vi "OCR_Determine Line bit array.vi"(8 "Error":errorcluster, 9 "Body Rect Array":T2[](array[typedef]), 11 "Border Removed":T6) -> (0 "Error Out":errorcluster, 3 "Text Out":T1[](array[typedef]), 4 "Status Of Each Line Out":bool[](array[boolean]))   [LabVIEW 2009]
uses:
  Controls/Array/Color Box Array_2D Icon Viewer.ctl
  Controls/Cluster/Cluster_Text Rect.ctl
  Controls/Cluster/Cluster_Region info.ctl
  Controls/Cluster/Cluster_Top Left position.ctl
  Controls/Cluster/Cluster_Text Color Set.ctl
  Controls/String_Picture/STRING_Line Display.ctl
  Controls/Cluster/Cluster_Bit array and line status.ctl
  Controls/String_Picture/String Char Normal.ctl
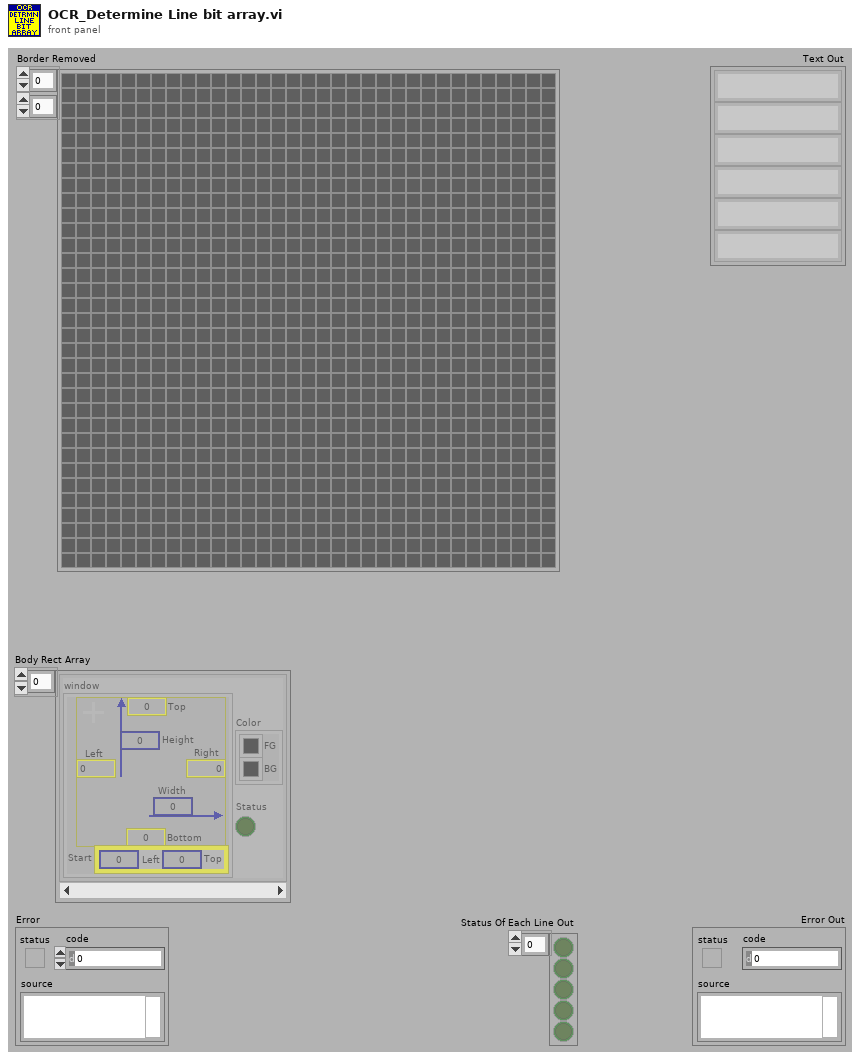
[diagram p1: front panel]
types:
  T1 = typedef "STRING_Line Display.ctl" = string
  T2 = typedef "Cluster_Text Rect.ctl" = cluster{"window":T3, "Color":T5, "Status":bool}
  T3 = typedef "Cluster_Region info.ctl" = cluster{"Left":i32, "Top":i32, "Right":i32, "Bottom":i32, "Width":u32, "Height":u32, "Start":T4}
  T4 = typedef "Cluster_Top Left position.ctl" = cluster{"Left":i32, "Top":i32}
  T5 = typedef "Cluster_Text Color Set.ctl" = cluster{"BG":u32, "FG":u32}
  T6 = typedef "Color Box Array_2D Icon Viewer.ctl" = u32[][]
  T7 = typedef "Cluster_Bit array and line status.ctl" = cluster{"Char Array":T8[], "Status":bool}
  T8 = typedef "String Char Normal.ctl" = string
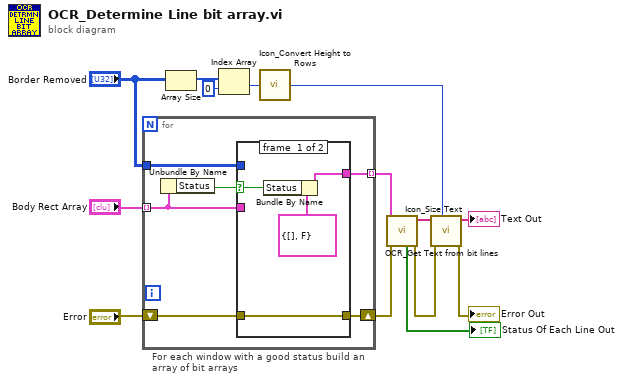
[diagram p0: block diagram]
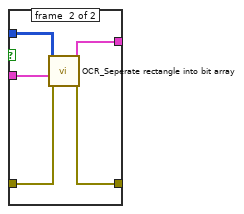
[diagram p2: hidden frame]
diagram:
  n1 = for "For each window with a good status build an array of bit arrays" {
    tunnel: [w17] -> w12 mode=indexing
    tunnel: "Body Rect Array" -> [w15] mode=indexing
    shift-right: [w19] -> w11
    shift-left: "Error" -> [w20]
    tunnel: "Border Removed" -> [w18]
    n2 = Unbundle By Name(w15) -> ("Status"=w16:bool)
    n3 = case shown="False" w16 {
      selector: w16 -> [w21 _]
      tunnel: w20 -> [w24 w29]
      tunnel: [w24 w28] -> w19
      tunnel: w18 -> [_ w27]
      tunnel: w15 -> [_ w26]
      tunnel: [w22 w25] -> w17
      frame #0 {
        n4 = Bundle By Name(cluster=T7 {"Char Array"=[], "Status"=FALSE} ("Bit Array Out"), "Status"=w21) -> (w22:T7)
      }
      frame #1 {
        n5 = call "OCR_Seperate rectangle into bit array.vi"("Error"=w29, "Text Rect."=w26, "2D Image"=w27) -> ("Error Out"=w28:errorcluster, "Bit Array Out"=w25:T7)  [unwired: 7 in]
      }
    }
  }
  n6 = Array Size(array="Border Removed") -> (size(s)=w10:i32[])
  n7 = Index Array(array=w10, index=0) -> (element=w8:i32)
  n8 = call "Icon_Convert Height to Rows.vi"("Height"=w8) -> ("Rows"=w7:u32)  [unwired: 4 in]
  n9 = call "OCR_Get Text from bit lines.vi"("Error"=w11, "Bit Line Array"=w12) -> ("Error Out"=w6:errorcluster, "Text Out"=w4:T1[], "Status Of Each Line Out"=→"Status Of Each Line Out":bool[])  [unwired: 7 in]
  n10 = call "Icon_Size Text.vi"("Rows"=w7, "Error"=w6, "Text"=w4) -> ("Error Out"=→"Error Out":errorcluster, "Text Out"=→"Text Out":T1[])  [unwired: 7 in]
